vi "Get VI Name.vi"(8 "error in (no error)":errorcluster, 11 "VI Refnum In (if empty use parrent name)":refnum<vi>) -> (0 "error out":errorcluster, 1 "VI Name without extension":string, 2 "VI Name":string)   [LabVIEW 2019]
doc: "Get VI Name."
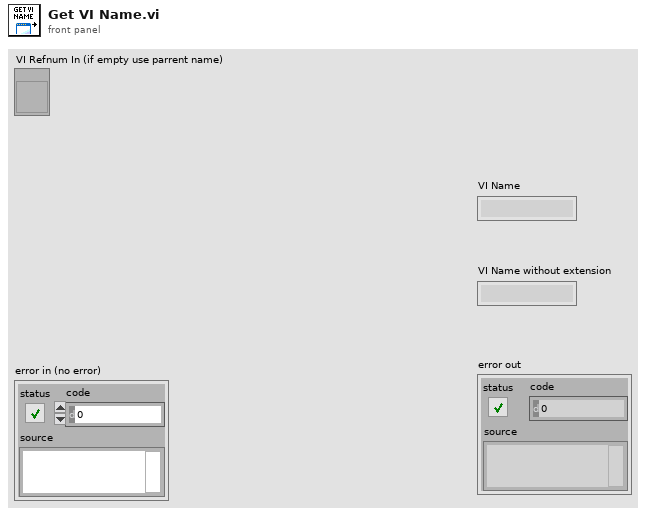
[diagram p1: front panel]
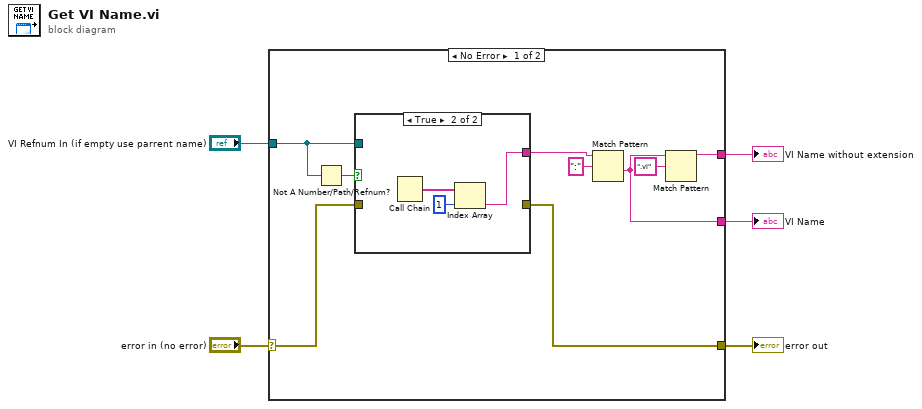
[diagram p0: block diagram]
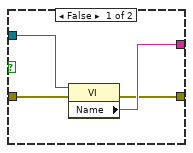
[diagram p2: hidden frame]
diagram:
  n1 = case shown="No Error" "error in (no error)" {
    selector: "error in (no error)" -> [w7 w22]
    tunnel: [w12 _] -> w2
    tunnel: "VI Refnum In (if empty use parrent name)" -> [w11 _]
    tunnel: [w10 _] -> w1
    tunnel: [w6 w22] -> w3
    frame No Error {
      n2 = Not A Number/Path/Refnum?(number/path/refnum=w11) -> (NaN/Path/Refnum?=w9:bool)
      n3 = case shown="True" w9 {
        tunnel: w11 -> [w18 _]
        tunnel: [w17 w19] -> w8
        tunnel: [w16 _] -> w6
        tunnel: w7 -> [w15 _]
        frame False {
          n4 = property class="VI"(reference=w18, error in=w15) -> (error out=w16:errorcluster, "Name"=w17:string)  [unwired: 1 out]
        }
        frame True {
          n5 = Call Chain() -> (call chain=w20:string[])
          n6 = Index Array(array=w20, index=1) -> (element=w19:string)
        }
      }
      n7 = Match Pattern(string=w8, regular expression=":" ("Regulärer Ausdruck")) -> (after substring=w10:string)  [unwired: 1 in, 3 out]
      n8 = Match Pattern(string=w10, regular expression=".vi" ("Regulärer Ausdruck")) -> (before substring=w12:string)  [unwired: 1 in, 3 out]
    }
    frame Error {
    }
  }
  "VI Name" <- w1
  "VI Name without extension" <- w2
  "error out" <- w3
